vi "writeCursorConfigMain.vi"(8 "error in (no error)":errorcluster, 11 "Cursor Locations":T1={"DC1"=200, "DC2"=250, "BG1"=10, "BG2"=100}) -> (0 "error out":errorcluster)   [LabVIEW 2020]
uses:
  <vilib>/Utility/config.llb/Write Key (I32).vi
  <vilib>/Utility/config.llb/NI_LVConfig.lvlib
panel:
  out "file path":path
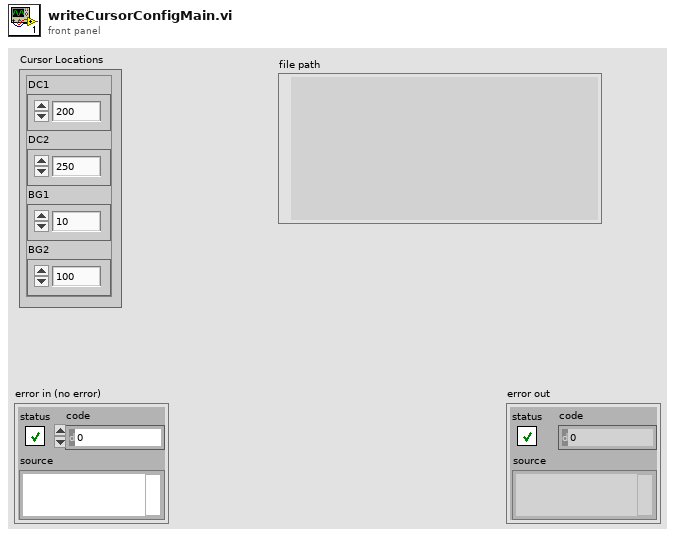
[diagram p1: front panel]
types:
  T1 = cluster{"DC1":i32, "DC2":i32, "BG1":i32, "BG2":i32}
  T2 = typedef "NI_LVConfig.lvlib/Config Data RefNum.ctl" = refnum<k1>
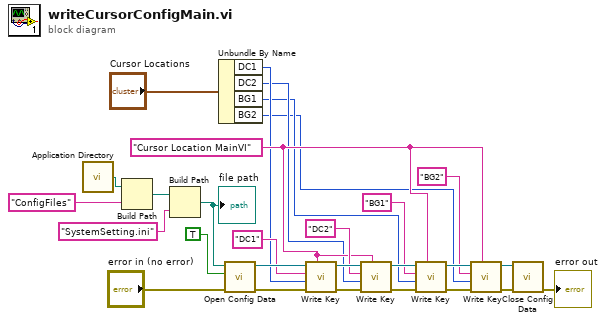
[diagram p0: block diagram]
diagram:
  w7 = "Cursor Location MainVI" ("section")
  n1 = call <vilib>:"Application Directory.vi"() -> ("Application Directory"=w26:path)
  n2 = Build Path(base path=w26, name or relative path="ConfigFiles") -> (appended path=w24:path)
  n3 = Build Path(base path=w24, name or relative path="SystemSetting.ini") -> (appended path=w22:path)
  "file path" <- w22
  n4 = Unbundle By Name("Cursor Locations") -> ("DC1"=w4:i32, "DC2"=w3:i32, "BG1"=w2:i32, "BG2"=w1:i32)
  n5 = call <vilib>:"Open Config Data.vi"("error in (no error)"="error in (no error)", "create file if necessary (T)"=TRUE, "configuration file path"=w22) -> ("error out"=w19:errorcluster, "refnum"=w21:T2)  [unwired: 6 in, 1 out]
  n6 = call-poly <vilib>:"Write Key.vi"("section"=w7, "error in (no error)"=w19, "value"=w4, "key"="DC1", "refnum"=w21) -> ("error out"=w17:errorcluster, "refnum out"=w18:T2)  [unwired: 4 in, 1 out]
  n7 = call-poly <vilib>:"Write Key.vi"("section"=w7, "error in (no error)"=w17, "value"=w3, "key"="DC2", "refnum"=w18) -> ("error out"=w14:errorcluster, "refnum out"=w15:T2)  [unwired: 4 in, 1 out]
  n8 = call-poly <vilib>:"Write Key.vi"("section"=w7, "error in (no error)"=w14, "value"=w2, "key"="BG1", "refnum"=w15) -> ("error out"=w10:errorcluster, "refnum out"=w12:T2)  [unwired: 4 in, 1 out]
  n9 = call-poly <vilib>:"Write Key.vi"("section"=w7, "error in (no error)"=w10, "value"=w1, "key"="BG2", "refnum"=w12) -> ("error out"=w5:errorcluster, "refnum out"=w6:T2)  [unwired: 4 in, 1 out]
  n10 = call <vilib>:"Close Config Data.vi"("error in (no error)"=w5, "refnum"=w6) -> ("error out"=→"error out":errorcluster)  [unwired: 8 in, 1 out]
